vi "Example 4 (Create FPGA Addon).vi"() -> ()   [LabVIEW 2018]
uses:
  <vilib>/addons/VeriStand Custom Device Scripting APIs/FPGA Addon/Scripting API.lvlibp
panel:
  out "error out":errorcluster
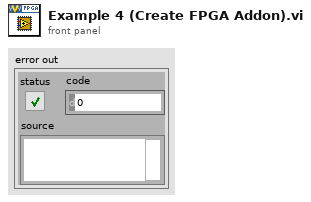
[diagram p1: front panel]
types:
  T1 = typedef "Scripting API.lvlibp/Custom Device API.lvlib/Custom Device Item Ref.ctl" = u64
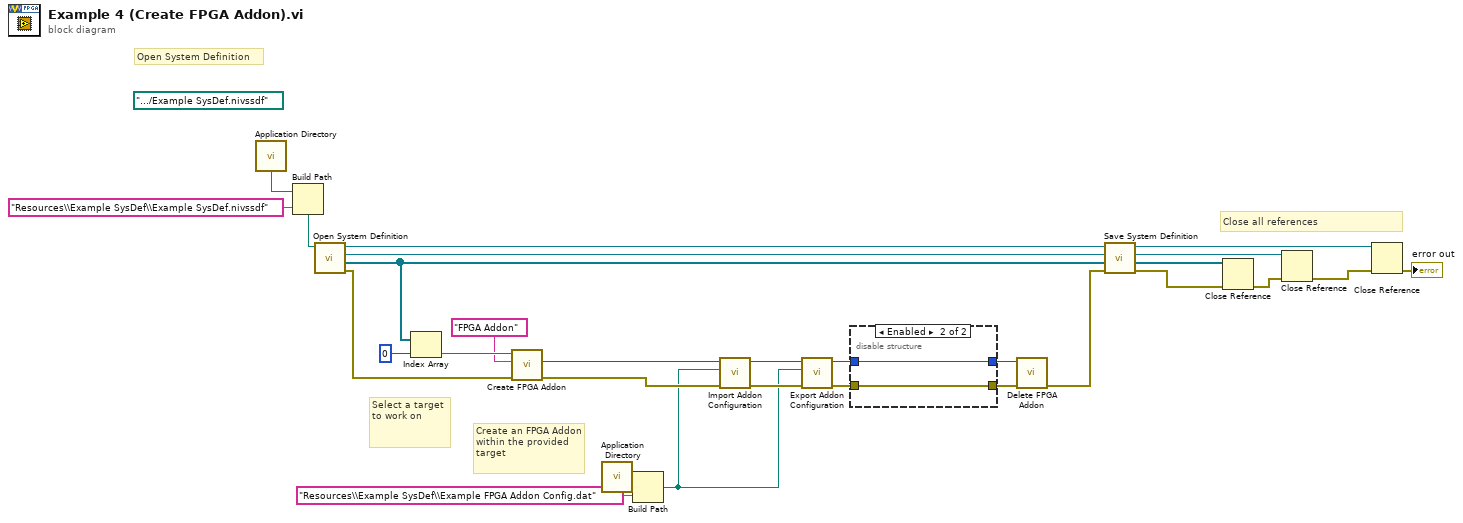
[diagram p0: block diagram]
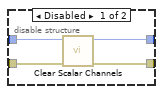
[diagram p2: hidden frame]
diagram:
  (unwired) path ".../Example SysDef.nivssdf" ("fpga bitfile path")
  # "Close all references"
  # "Create an FPGA Addon within the provided target"
  # "Select a target to work on"
  # "Open System Definition"
  n1 = call <vilib>:"Application Directory.vi"() -> ("Application Directory"=w22:path)
  n2 = Build Path(base path=w22, name or relative path="Resources\\Example SysDef\\Example SysDef.nivssdf") -> (appended path=w20:path)
  n3 = call "Open System Definition.vi"("System Definition File"=w20) -> ("error out"=w9:errorcluster, "targets refnums"=w25:refnum<k24>[], "root refnum"=w26:refnum<k24>, "system definition refnum"=w18:refnum<k24>)  [unwired: 7 in]
  n4 = Index Array(array=w25, index=0) -> (element=w14:refnum<k24>)
  n5 = call <vilib>:"Create FPGA Addon.vi"("error in (no error)"=w9, "FPGA Addon name"="FPGA Addon" ("fpga addon name"), "target in"=w14) -> ("error out"=w10:errorcluster, "FPGA Addon refnum"=w12:T1)  [unwired: 6 in, 1 out]
  n6 = call <vilib>:"Application Directory.vi"() -> ("Application Directory"=w15:path)
  n7 = Build Path(base path=w15, name or relative path="Resources\\Example SysDef\\Example FPGA Addon Config.dat") -> (appended path=w6:path)
  n8 = call <vilib>:"Import Addon Configuration.vi"("error in (no error)"=w10, "configuration file path"=w6, "FPGA Addon refnum in"=w12) -> ("error out"=w8:errorcluster, "FPGA Addon refnum out"=w7:T1)  [unwired: 7 in]
  n9 = call <vilib>:"Export Addon Configuration.vi"("error in (no error)"=w8, "export file path"=w6, "FPGA Addon refnum in"=w7) -> ("error out"=w5:errorcluster, "FPGA Addon refnum out"=w4:T1)  [unwired: 7 in]
  n10 = disable-structure shown="Enabled" {
    disable-tunnel: w5 -> [w31 w33]
    disable-tunnel: [w28 w33] -> w3
    disable-tunnel: w4 -> [w30 w32]
    disable-tunnel: [w29 w32] -> w2
    frame Disabled {
      n11 = call <vilib>:"Clear Scalar Channels.vi"("error in (no error)"=w31, "FPGA Addon refnum in"=w30) -> ("error out"=w28:errorcluster, "FPGA Addon refnum out"=w29:T1)  [unwired: 8 in]
    }
    frame Enabled {
    }
  }
  n12 = call <vilib>:"Delete FPGA Addon.vi"("error in (no error)"=w3, "FPGA Addon refnum"=w2) -> ("error out"=w1:errorcluster)  [unwired: 8 in, 1 out]
  n13 = call "Save System Definition.vi"("error in (no error)"=w1, ".NET Refnum in"=w18) -> ("error out"=w16:errorcluster, ".NET Refnum out"=w17:refnum<k24>)  [unwired: 8 in]
  n14 = Close Reference(reference=w25, error in (no error)=w16) -> (error out=w24:errorcluster)
  n15 = Close Reference(reference=w26, error in (no error)=w24) -> (error out=w23:errorcluster)
  n16 = Close Reference(reference=w17, error in (no error)=w23) -> (error out=→"error out":errorcluster)
